vi "6.1.vi"   [LabVIEW 2017]
types:
  T1 = enum16{"open", "replace", "create", "open or create", "replace or create", "replace or create with confirmation"}
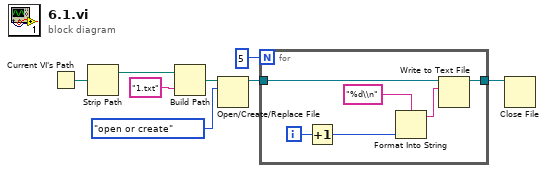
[diagram p0: block diagram]
diagram:
  n1 = Current VI's Path() -> (path=w8:path)
  n2 = Strip Path(path=w8) -> (stripped path=w7:path)  [unwired: 1 out]
  n3 = Build Path(base path=w7, name or relative path="1.txt" ("名称或相对路径")) -> (appended path=w4:path)
  n4 = Open/Create/Replace File(file path (use dialog)=w4, operation (0:open)=T1."open or create" ("操作(0:open)")) -> (refnum out=w3:refnum<file>)  [unwired: 4 in, 2 out]
  n5 = for {
    N: 5 -> [_]
    tunnel: w3 -> [w13]
    tunnel: [w9] -> w2
    i -> [w14]
    n6 = Increment(x=w14) -> (x+1=w11:i32)
    n7 = Format Into String(format string="%d\\n" ("格式字符串"), w11) -> (resulting string=w10:string)  [unwired: 2 in, 1 out]
    n8 = Write to Text File(file (use dialog)=w13, text=w10) -> (refnum out=w9:refnum<file>)  [unwired: 2 in, 2 out]
  }
  n9 = Close File(refnum=w2) -> ()  [unwired: 1 in, 2 out]
